vi "计算三角形垂心.vi"(8 "Error In":errorcluster caption="错误输入", 11 "三角形":T1) -> (0 "Error Out":errorcluster caption="错误输出", 3 "垂心":T2)   [LabVIEW 2012, in "几何工具.lvlib"]
uses:
  <vilib>/Utility/miscctls.llb/LVPointDoubleTypeDef.ctl
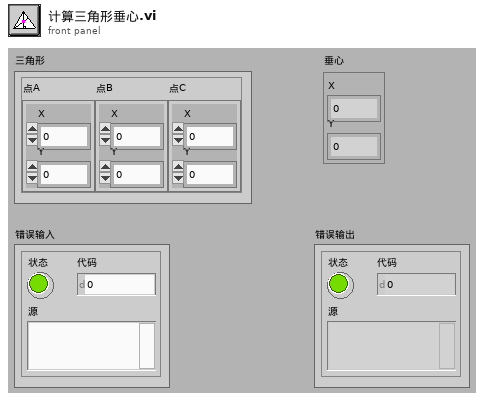
[diagram p1: front panel]
types:
  T1 = typedef "几何工具.lvlib/三角形.ctl" = cluster{"点A":T2, "点B":T2, "点C":T2}
  T2 = typedef "LVPointDoubleTypeDef.ctl" = cluster{"X":dbl, "Y":dbl}
  T3 = typedef "几何工具.lvlib/斜率与截距.ctl" = cluster{"斜率":dbl, "截距":dbl}
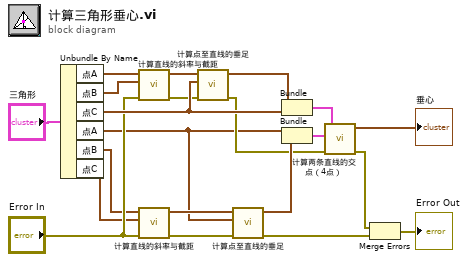
[diagram p0: block diagram]
diagram:
  n1 = Unbundle By Name("三角形") -> ("点A"=w14:T2, "点B"=w18:T2, "点C"=w16:T2, "点A"=w4:T2, "点B"=w3:T2, "点C"=w2:T2)
  n2 = call "计算直线的斜率与截距.vi"("Error In"="Error In", "点B"=w18, "点A"=w14) -> ("Error Out"=w9:errorcluster, "斜率与截距"=w19:T3)  [unwired: 7 in]
  n3 = call "计算直线的斜率与截距.vi"("Error In"="Error In", "点B"=w2, "点A"=w3) -> ("Error Out"=w11:errorcluster, "斜率与截距"=w20:T3)  [unwired: 7 in]
  n4 = call "计算点至直线的垂足.vi"("Error In"=w9, "Point"=w16, "直线"=w19) -> ("Error Out"=w8:errorcluster, "垂足点"=w17:T2)  [unwired: 7 in]
  n5 = call "计算点至直线的垂足.vi"("Error In"=w11, "Point"=w4, "直线"=w20) -> ("Error Out"=w6:errorcluster, "垂足点"=w15:T2)  [unwired: 7 in]
  n6 = Bundle("垂足点"=w17, "点C"=w16) -> (w13:cluster{"垂足点":T2, "点C":T2})  [unwired: 1 in]
  n7 = Bundle("点A"=w4, "垂足点"=w15) -> (w1:cluster{"点A":T2, "垂足点":T2})  [unwired: 1 in]
  n8 = call "计算两条直线的交点（4点）.vi"("Error In"=w8, "直线B"=w1, "直线A"=w13) -> ("Error Out"=w7:errorcluster, "交点"=→"垂心":T2)  [unwired: 7 in]
  n9 = Merge Errors(w7, w6) -> (→"Error Out":errorcluster)
